vi "Finish Acquisition.vi"(9 "Logging Cluster":T1 {"Exp params"."TSFrames" min=1 step=1; "Exp params"."TSfps" min=0.001 max=90.0 step=0.001 format="%_4g"}) -> ()   [LabVIEW 2020]
uses:
  _controls/Logging Cluster.ctl
  _controls/Exp Params.ctl
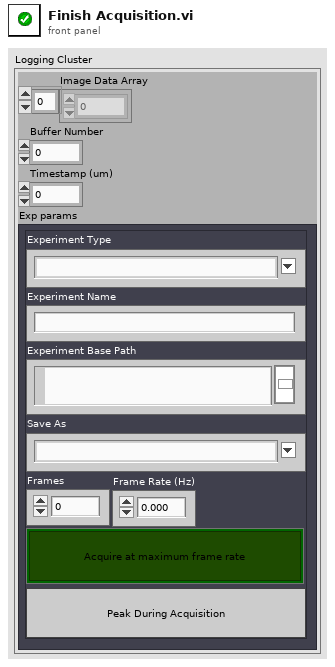
[diagram p1: front panel]
types:
  T1 = typedef "Logging Cluster.ctl" = cluster{"Image Data Array":u8[], "Buffer Number":i32, "Timestamp (um)":u64, "Exp params":T2}
  T2 = typedef "Exp Params.ctl" = cluster{"Experiment Type":string, "Experiment Name":string, "ExpPath":path, "Save As":string, "TSFrames":i32, "TSfps":dbl, "Streaming":bool, "tdms ref":refnum<k34>, "frame #":i64, "Full Path":path, "PeakOnQueue":bool}
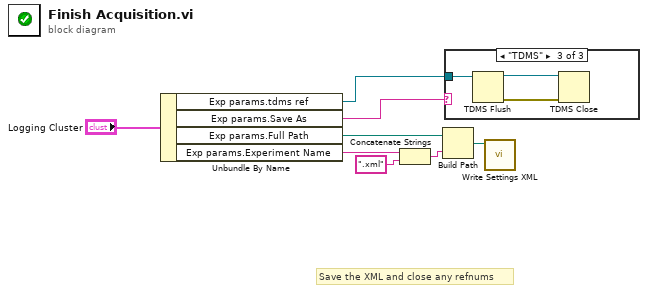
[diagram p0: block diagram]
diagram:
  # "Save the XML and close any refnums"
  n1 = Unbundle By Name("Logging Cluster") -> ("Exp params.tdms ref"=w1:refnum<k34>, "Exp params.Save As"=w2:string, "Exp params.Full Path"=w3:path, "Exp params.Experiment Name"=w5:string)
  n2 = Concatenate Strings(w5, ".xml" ("string")) -> (w7:string)
  n3 = Build Path(base path=w3, name or relative path=w7) -> (appended path=w4:path)
  n4 = case shown="\"TDMS\"" w2 {
    tunnel: w1 -> [_ _ w11]
    frame "TIFF", Default {
    }
    frame "RAW" {
    }
    frame "TDMS" {
      n5 = TDMS Flush(7:w11) -> (0:w9:errorcluster, 3:w10:refnum<k34>)  [unwired: 1 in]
      n6 = TDMS Close(8:w9, 11:w10) -> ()  [unwired: 2 out]
    }
  }
  n7 = call "Write Settings XML.vi"("path"=w4) -> ()  [unwired: 9 in, 2 out]
